vi "Stop Scheduled Polling.vi"(8 "error in":errorcluster, 11 "Instruments in":refnum<class "Instruments.lvclass">) -> (0 "error out":errorcluster, 3 "Instruments out":refnum<class "Instruments.lvclass">)   [LabVIEW 2023, in "Instruments.lvlib" / "Instruments.lvclass"]
uses:
  Library/Instruments.lvclass
  Library/Instruments.lvclass/Instruments.ctl
  builds/Engine/Actor Framework.lvlibp/1abvi3w/vi.lib/ActorFramework/Time-Delayed Send Message/Time-Delay Override Options.ctl
  builds/Engine/Actor Framework.lvlibp
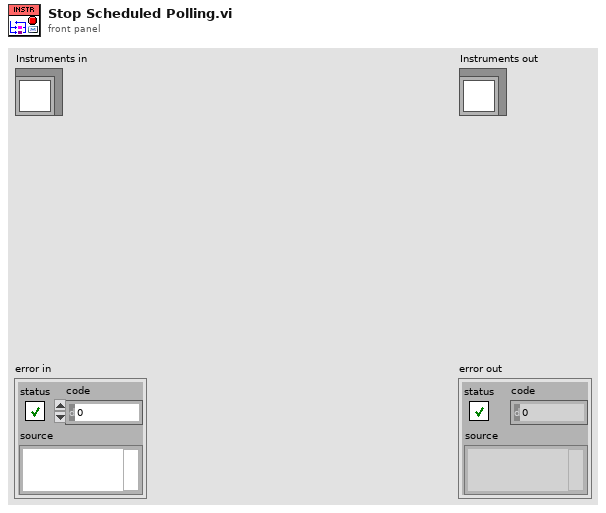
[diagram p1: front panel]
types:
  T1 = typedef "Actor Framework.lvlibp/Time-Delay Override Options.ctl" = enum16{"Send next copy now", "Skip next scheduled copy", "Send next copy now and stop all further copies", "Stop all further copies"}
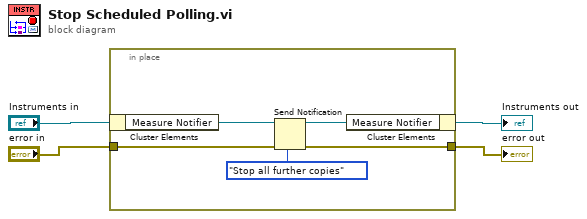
[diagram p0: block diagram]
diagram:
  n1 = in-place {
    in-place-border: [w6] -> w2
    in-place-border: "error in" -> [w5]
    n2 = in-place-cluster #1("Instruments in") -> ("Measure Notifier"=w9:refnum<notifier>)
    n3 = Send Notification(notification=Time-Delay_Override_Options."Stop all further copies", notifier=w9, error in (no error)=w5) -> (notifier out=w8:refnum<notifier>, error out=w6:errorcluster)
    n4 = in-place-cluster #1("Measure Notifier"=w8) -> (→"Instruments out":refnum<class "Instruments.lvclass">)
  }
  "error out" <- w2
